vi "LV RT Doc - Instantiate with Ref.vi"(0 "VI Refnum":refnum<vi>, 11 "error in (no error)":errorcluster) -> (4 "LV RT":refnum<class "LV RT.lvclass">, 15 "error out":errorcluster)   [LabVIEW 2016, in "LV RT.lvclass"]
uses:
  LV RT.lvclass
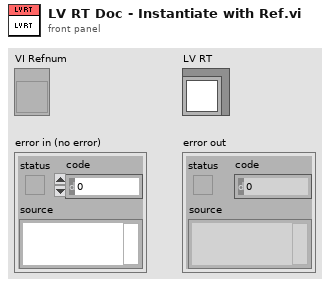
[diagram p1: front panel]
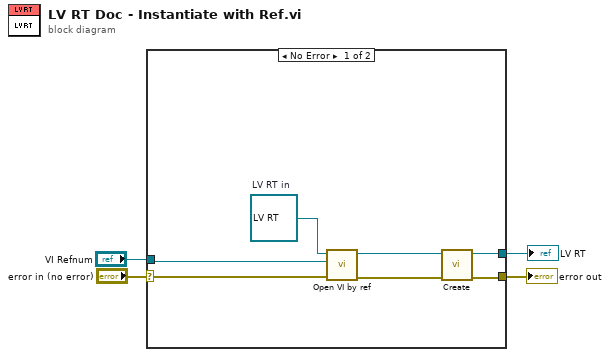
[diagram p0: block diagram]
diagram:
  n1 = case shown="No Error" "error in (no error)" {
    selector: "error in (no error)" -> [w8 w12]
    tunnel: [w6 w12] -> w3
    tunnel: "VI Refnum" -> [w7 _]
    tunnel: [w5 _] -> w1
    frame No Error {
      w11 = refnum<class "LV RT.lvclass"> refnum  # LV RT in
      n2 = call "Open VI by ref.vi"("error in (no error)"=w8, "reference"=w7, "LV RT in"=w11) -> ("error out"=w10:errorcluster, "LV RT out"=w9:refnum<class "LV RT.lvclass">)  [unwired: 7 in]
      n3 = call-dynamic "Create.vi"("error in (no error)"=w10, "Document in"=w9) -> ("error out"=w6:errorcluster, "Document out"=w5:refnum<class "LV RT.lvclass">)  [unwired: 8 in]
    }
    frame Error {
    }
  }
  "error out" <- w3
  "LV RT" <- w1
